vi "Action Status to Text.vi"(1 "PSU Act Stat":T1) -> (0 "Status:":string)   [LabVIEW 2019, in "Instrument.OxfordVRM.lvclass"]
uses:
  Instrument.OxfordVRM.lvclass
  <instrlib>/Mercury iXX/Public/Libraries/Magnet/Controls/PSU Actions.ctl
  <instrlib>/Mercury iXX/Public/Libraries/Magnet.lvlib
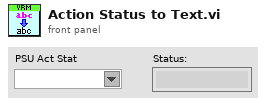
[diagram p1: front panel]
types:
  T1 = typedef "Mercury iXX.lvlib/Magnet.lvlib/PSU Actions.ctl" = string
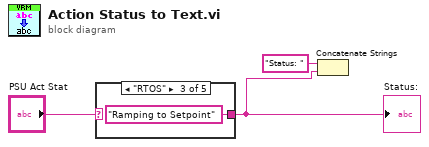
[diagram p0: block diagram]
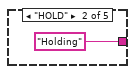
[diagram p3: hidden frame]
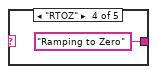
[diagram p4: hidden frame]
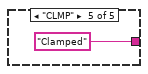
[diagram p5: hidden frame]
diagram:
  n1 = case shown="\"RTOS\"" "PSU Act Stat" {
    selector: "PSU Act Stat" -> [w4 _ _ _ _]
    tunnel: [w4 "Holding" "Ramping to Setpoint" "Ramping to Zero" "Clamped"] -> w1
    frame Default {
    }
    frame "HOLD" {
    }
    frame "RTOS" {
    }
    frame "RTOZ" {
    }
    frame "CLMP" {
    }
  }
  "Status:" <- w1
  n2 = Concatenate Strings("Status: " ("string"), w1) -> ()  [unwired: 1 out]
